vi "M0 Smart Grid.vi"(11 "EV3 in":T1) -> (3 "EV3 out":T1)   [LabVIEW 2016]
uses:
  <vilib>/NXT/Subs/LVHSConnector.ctl
  <vilib>/NXT/LegoClasses/BrickReference/BrickReference.lvclass
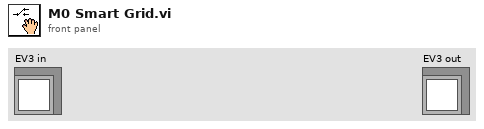
[diagram p1: front panel]
types:
  T1 = typedef "LVHSConnector.ctl" = refnum<class "BrickReference.lvclass">
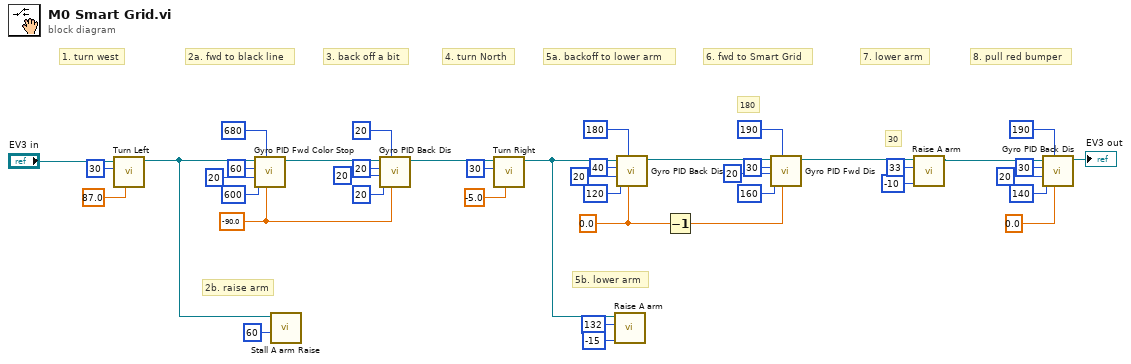
[diagram p0: block diagram]
diagram:
  w25 = sgl 0.0 ("Target angle")
  w19 = sgl -90.0 ("Target angle")
  # "180"
  # "30"
  # "8. pull red bumper"
  # "7. lower arm"
  # "6. fwd to Smart Grid"
  # "5b. lower arm"
  # "5a. backoff to lower arm"
  # "4. turn North"
  # "3. back off a bit"
  # "2b. raise arm"
  # "2a. fwd to black line"
  # "1. turn west"
  n1 = call "Turn Left.vi"("Turning angle"=sgl 87.0, "Motor B (right)"=i8 30, "EV3 in"="EV3 in") -> ("EV3 out"=w36:T1)  [unwired: 8 in]
  n2 = call "Gyro PID Fwd Color Stop.vi"("Target angle"=w19, "Threshold to Color"=680, "Threshold to slow"=600, "Min. speed"=20, "Max. speed"=60, "EV3 in"=w36) -> ("EV3 out"=w20:T1)  [unwired: 5 in]
  n3 = call "Stall A arm Raise.vi"("Power"=i8 60, "NXT/EV3"=w36) -> ()  [unwired: 9 in, 1 out]
  n4 = call "Gyro PID Back Dis.vi"("Target angle"=w19, "Threshold to stop"=20, "Threshold to slow"=20, "Min. speed"=20, "Max. speed"=20, "EV3 in"=w20) -> ("EV3 out"=w18:T1)  [unwired: 5 in]
  n5 = call "Turn Right.vi"("Turning angle"=sgl -5.0, "Motor B (right)"=i8 30, "EV3 in"=w18) -> ("EV3 out"=w6:T1)  [unwired: 8 in]
  n6 = call "Raise A arm.vi"("Power"=i8 -15, "Rotation"=132, "EV3 in"=w6) -> ()  [unwired: 8 in, 1 out]
  n7 = call "Gyro PID Back Dis.vi"("Target angle"=w25, "Threshold to stop"=180, "Threshold to slow"=120, "Min. speed"=20, "Max. speed"=40, "EV3 in"=w6) -> ("EV3 out"=w5:T1)  [unwired: 5 in]
  n8 = Decrement(x=w25) -> (x-1=w1:sgl)
  n9 = call "Gyro PID Fwd Dis.vi"("Target angle"=w1, "Threshold to stop"=190, "Threshold to slow"=160, "Min. speed"=20, "Max. speed"=30, "EV3 in"=w5) -> ("EV3 out"=w15:T1)  [unwired: 5 in]
  n10 = call "Raise A arm.vi"("Power"=i8 -10, "Rotation"=33, "EV3 in"=w15) -> ("EV3 out"=w9:T1)  [unwired: 8 in]
  n11 = call "Gyro PID Back Dis.vi"("Target angle"=sgl 0.0, "Threshold to stop"=190, "Threshold to slow"=140, "Min. speed"=20, "Max. speed"=30, "EV3 in"=w9) -> ("EV3 out"=→"EV3 out":T1)  [unwired: 5 in]
